vi "Get Installed 7z.vi"(8 "error in (no error)":errorcluster) -> (0 "error out":errorcluster, 3 "Application Path":string)   [LabVIEW 2019, in "PostBuildSupport.lvclass"]
uses:
  PostBuildSupport.lvclass
  <vilib>/registry/registry.llb/Registry RtKey.ctl
  <vilib>/registry/registry.llb/Registry View.ctl
  <vilib>/registry/registry.llb/Registry SAM.ctl
  <vilib>/registry/registry.llb/Read Registry Value Simple STR.vi
  <vilib>/Utility/error.llb/Error Cluster From Error Code.vi
  <vilib>/ErrorRing/Error Ring.xnode
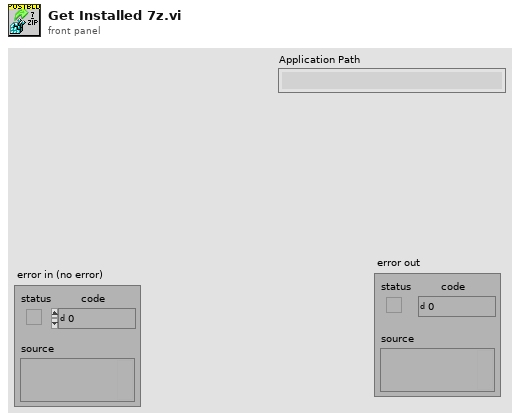
[diagram p1: front panel]
types:
  T1 = typedef "Registry RtKey.ctl" = enum32{"HKEY_CLASSES_ROOT", "HKEY_CURRENT_USER", "HKEY_LOCAL_MACHINE", "HKEY_USERS", "HKEY_PERFORMANCE_DATA", "HKEY_CURRENT_CONFIG", "HKEY_DYN_DATA"}
  T2 = typedef "Registry SAM.ctl" = enum32{"KEY_QUERY_VALUE", "KEY_SET_VALUE", "KEY_CREATE_SUB_KEY", "KEY_ENUMERATE_SUB_KEYS", "KEY_NOTIFY", "KEY_CREATE_LINK", "KEY_READ", "KEY_WRITE", "KEY_ALL_ACCESS", "KEY_READ | KEY_WRITE"}
  T3 = typedef "Registry View.ctl" = u16
  T4 = typedef "Registry refnum.ctl" = refnum<k1>
  T5 = cluster{"numSubKeys":i32, "maxSubKeyLen":i32, "maxSubKeyClassLen":i32}
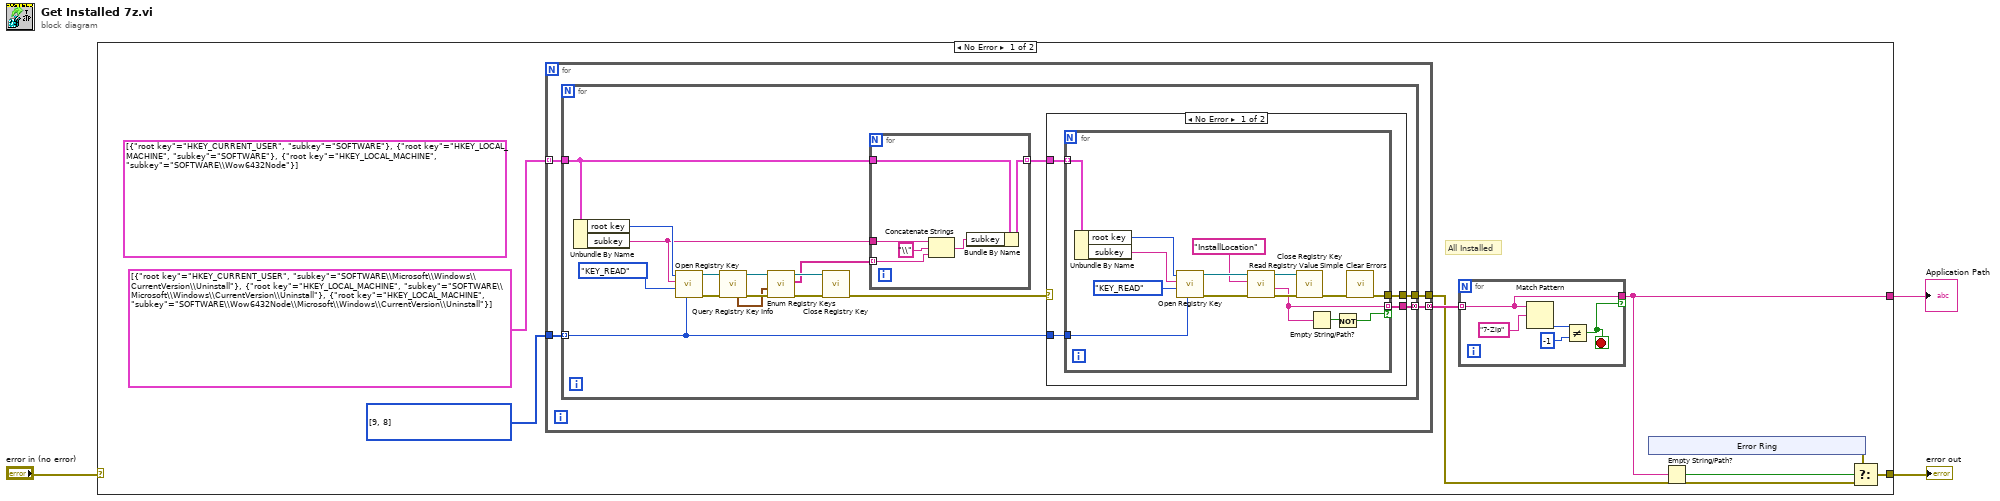
[diagram p0: block diagram]
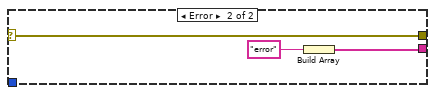
[diagram p2: hidden frame]
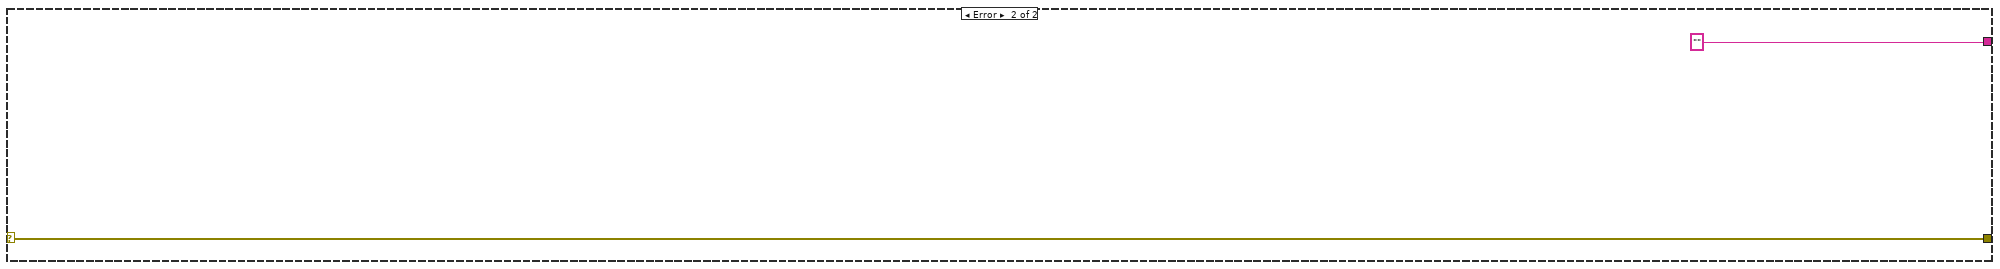
[diagram p3: hidden frame]
diagram:
  n1 = case shown="No Error" "error in (no error)" {
    selector: "error in (no error)" -> [_ w71]
    tunnel: [w7 "" ("String/Binary data")] -> w3
    tunnel: [w5 w71] -> w1
    frame No Error {
      w10 = T3[] [9, 8] items=["Default"=0, "KEY_WOW64_64KEY"=8, "KEY_WOW64_32KEY"=9] ("registry view")
      (unwired) cluster{"root key":T1, "subkey":string}[] [{"root key"=enum."HKEY_CURRENT_USER", "subkey"="SOFTWARE"}, {"root key"=enum."HKEY_LOCAL_MACHINE", "subkey"="SOFTWARE"}, {"root key"=enum."HKEY_LOCAL_MACHINE", "subkey"="SOFTWARE\\Wow6432Node"}]
      # "All Installed"
      n2 = for {
        tunnel: [w24] -> w9 mode=concatenating
        tunnel: cluster{"root key":T1, "subkey":string}[] [{"root key"=enum."HKEY_CURRENT_USER", "subkey"="SOFTWARE\\Microsoft\\Windows\\CurrentVersion\\Uninstall"}, {"root key"=enum."HKEY_LOCAL_MACHINE", "subkey"="SOFTWARE\\Microsoft\\Windows\\CurrentVersion\\Uninstall"}, {"root key"=enum."HKEY_LOCAL_MACHINE", "subkey"="SOFTWARE\\Wow6432Node\\Microsoft\\Windows\\CurrentVersion\\Uninstall"}] -> [w23] mode=indexing
        tunnel: w10 -> [w22]
        tunnel: [w21] -> w4
        n3 = for {
          tunnel: w23 -> [w34]
          tunnel: [w31] -> w24 mode=concatenating
          tunnel: w22 -> [w26] mode=indexing
          tunnel: [w25] -> w21
          n4 = Unbundle By Name(w34) -> ("root key"=w33:T1, "subkey"=w32:string)
          n5 = call <vilib>:"Open Registry Key.vi"("registry view"=w26, "security access mask (KEY_READ | KEY_WRITE)"=Registry_SAM."KEY_READ", "subkey"=w32, "root key (HKEY_LOCAL_MACHINE)"=w33) -> ("error out"=w39:errorcluster, "refnum out"=w35:T4)  [unwired: 6 in]
          n6 = call <vilib>:"Query Registry Key Info.vi"("error in (no error)"=w39, "refnum"=w35) -> ("error out"=w37:errorcluster, "refnum out"=w38:T4, "subkey info"=w27:T5)  [unwired: 5 in, 2 out]
          n7 = call <vilib>:"Enum Registry Keys.vi"("error in (no error)"=w37, "subkey info"=w27, "refnum"=w38) -> ("error out"=w40:errorcluster, "subkeys"=w28:string[], "refnum out"=w41:T4)  [unwired: 6 in]
          n8 = call <vilib>:"Close Registry Key.vi"("error in (no error)"=w40, "refnum"=w41) -> ("error out"=w30:errorcluster)  [unwired: 5 in]
          n9 = for {
            tunnel: w32 -> [w66]
            tunnel: w28 -> [w65] mode=indexing
            tunnel: w34 -> [w69]
            tunnel: [w68] -> w29 mode=indexing
            n10 = Concatenate Strings(w66, "\\" ("string"), w65) -> (w64:string)
            n11 = Bundle By Name(cluster=w69, "subkey"=w64) -> (w68:cluster{"root key":T1, "subkey":string})
          }
          n12 = case shown="No Error" w30 {
            selector: w30 -> [_ w62]
            tunnel: w29 -> [w45 _]
            tunnel: [w44 w61] -> w31
            tunnel: w26 -> [w43 _]
            tunnel: [w42 w62] -> w25
            frame No Error {
              n13 = for {
                tunnel: w45 -> [w54] mode=indexing
                tunnel: [w52] -> w44 mode=indexing if=w48
                tunnel: w43 -> [w49]
                tunnel: [w46] -> w42
                n14 = Unbundle By Name(w54) -> ("root key"=w59:T1, "subkey"=w50:string)
                n15 = call <vilib>:"Open Registry Key.vi"("registry view"=w49, "security access mask (KEY_READ | KEY_WRITE)"=Registry_SAM."KEY_READ", "subkey"=w50, "root key (HKEY_LOCAL_MACHINE)"=w59) -> ("error out"=w57:errorcluster, "refnum out"=w58:T4)  [unwired: 6 in]
                n16 = call-poly <vilib>:"Read Registry Value Simple.vi"("error in (no error)"=w57, "value"="InstallLocation", "refnum"=w58) -> ("error out"=w56:errorcluster, "String/Binary data"=w52:string, "refnum out"=w55:T4)  [unwired: 3 in, 1 out]
                n17 = call <vilib>:"Close Registry Key.vi"("error in (no error)"=w56, "refnum"=w55) -> ("error out"=w47:errorcluster)  [unwired: 5 in]
                n18 = Empty String/Path?(string/path=w52) -> (empty?=w51:bool)
                n19 = Not(x=w51) -> (.not. x?=w48:bool)
                n20 = call <vilib>:"Clear Errors.vi"("error in (no error)"=w47) -> ("error out"=w46:errorcluster)  [unwired: 5 in, 1 out]
              }
            }
            frame Error {
              n21 = Build Array("error") -> (w61:string[])
            }
          }
        }
      }
      n22 = for {
        tunnel: w9 -> [w17] mode=indexing
        tunnel: [w17] -> w7 if=w16
        stop <- w16 stop-if-true
        n23 = Match Pattern(string=w17, regular expression="7-Zip") -> (offset past match=w19:i32)  [unwired: 1 in, 3 out]
        n24 = Not Equal?(x=w19, y=-1) -> (x != y?=w16:bool)
      }
      n25 = xnode "Error Ring"() -> ("error out"=w6:errorcluster)
      n26 = Empty String/Path?(string/path=w7) -> (empty?=w8:bool)
      n27 = Select(t=w6, s=w8, f=w4) -> (s? t:f=w5:errorcluster)
    }
    frame Error {
    }
  }
  "Application Path" <- w3
  "error out" <- w1
